vi "CloseImaq.vi"(1 "error in (no error)":errorcluster, 2 "IMAQ Session In":refnum<k11>) -> (0 "error out":errorcluster)   [LabVIEW 2010]
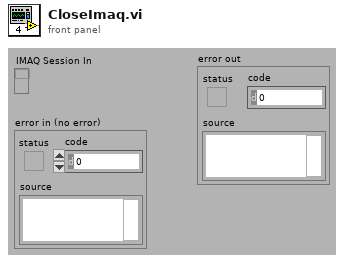
[diagram p1: front panel]
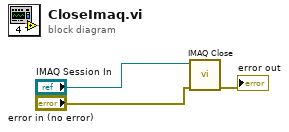
[diagram p0: block diagram]
diagram:
  n1 = call <vilib>:"IMAQ Close.vi"("error in (no error)"="error in (no error)", "IMAQ Session In"="IMAQ Session In") -> ("error out"=→"error out":errorcluster)  [unwired: 9 in]
